vi "Close.vi"(8 "error in (no error)":errorcluster, 11 "IMAQ Camera in":refnum<class "IMAQ Camera.lvclass">) -> (0 "error out":errorcluster, 3 "IMAQ Camera out":refnum<class "IMAQ Camera.lvclass">)   [LabVIEW 2011, in "IMAQ Camera.lvclass"]
uses:
  IMAQ Camera.lvclass
  IMAQ Camera.lvclass/IMAQ Camera.ctl
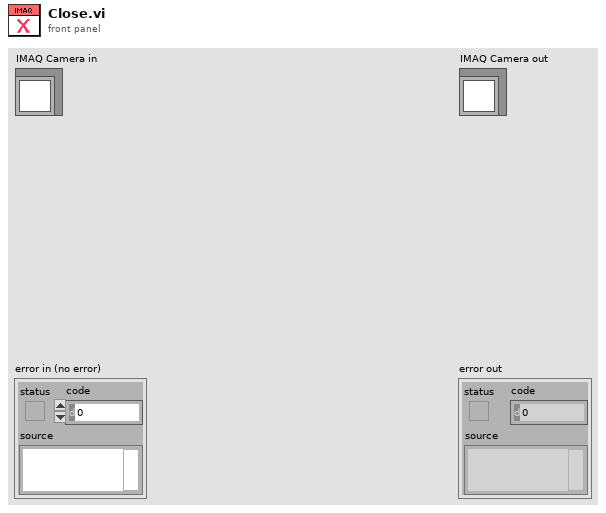
[diagram p1: front panel]
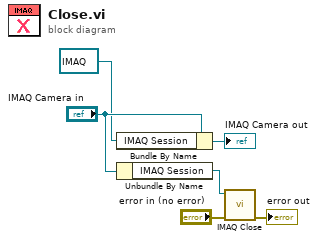
[diagram p0: block diagram]
diagram:
  n1 = Bundle By Name(cluster="IMAQ Camera in", "IMAQ Session"=refnum<k11> refnum) -> (→"IMAQ Camera out":refnum<class "IMAQ Camera.lvclass">)
  n2 = Unbundle By Name("IMAQ Camera in") -> ("IMAQ Session"=w6:refnum<k11>)
  n3 = call <vilib>:"IMAQ Close.vi"("error in (no error)"="error in (no error)", "IMAQ Session In"=w6) -> ("error out"=→"error out":errorcluster)  [unwired: 9 in]
